vi "Read Memory Data.vi"(8 "error in (no error)":errorcluster, 10 "Read Count (1)":i32=1 min=0 max=9999 format="%#.6g", 11 "VISA resource name":refnum<visa-resource-name>) -> (0 "error out":errorcluster, 1 "Measurements":string, 3 "VISA resource name out":refnum<visa-resource-name>)   [LabVIEW 2017, in "ADCMT7451_ADC.lvlib"]
doc: "This VI read measurements from memory."
uses:
  ADCMT7451_ADC.lvlib
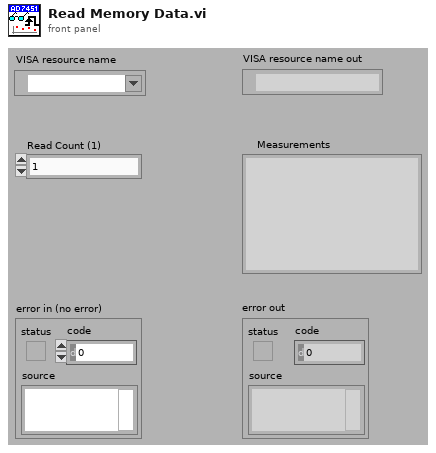
[diagram p1: front panel]
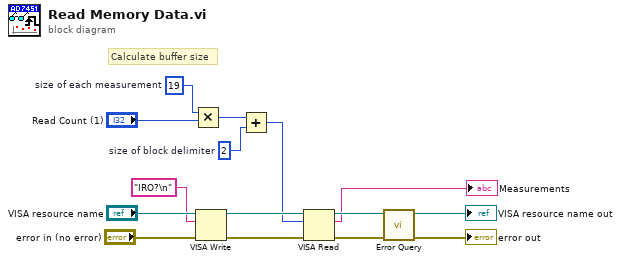
[diagram p0: block diagram]
diagram:
  w1 = 2  # size of block delimiter
  w7 = 19  # size of each measurement
  # "Calculate buffer size"
  n1 = Multiply(x=w7, y="Read Count (1)") -> (x*y=w6:i32)
  n2 = VISA Write(VISA resource name="VISA resource name", write buffer="IRO?\n", error in (no error)="error in (no error)") -> (VISA resource name out=w12:refnum<visa-resource-name>, error out=w13:errorcluster)  [unwired: 1 out]
  n3 = Add(x=w6, y=w1) -> (x+y=w5:i32)
  n4 = VISA Read(VISA resource name=w12, byte count=w5, error in (no error)=w13) -> (VISA resource name out=w15:refnum<visa-resource-name>, read buffer=→"Measurements":string, error out=w14:errorcluster)  [unwired: 1 out]
  n5 = call "Error Query.vi"("error in (no error)"=w14, "VISA resource name"=w15) -> ("error out"=→"error out":errorcluster, "VISA resource name out"=→"VISA resource name out":refnum<visa-resource-name>)  [unwired: 6 in, 2 out]
